vi "Client Input Test.vi"() -> (0 "error out":errorcluster, 2 "Pass?":bool)   [LabVIEW 2013, in "OPC UA Client Tests.lvlib"]
doc: "Test input override for OPC UA Client module."
uses:
  OPC UA Client Tests.lvlib
  <vilib>/NI/Tag Bus Module Framework/channel/channel classification.ctl
  module/execution/OPC UA Client runtime.lvclass
  module/execution/OPC UA Client runtime.lvclass/OPC UA Client runtime.ctl
  <vilib>/NI/Tag Bus Module Framework/channel/TBM channel.lvclass
panel:
  out "Individual Results":bool[](array[boolean])
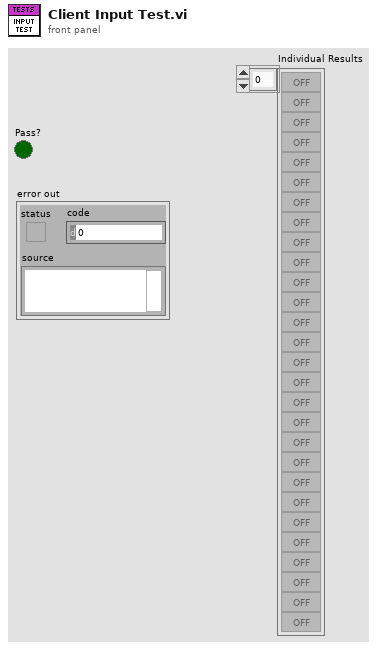
[diagram p1: front panel]
types:
  T1 = typedef "TBM channel.lvclass/channel classification.ctl" = enum16{"input data", "output data", "processing parameter", "processing result"}
  T2 = typedef "TBM channel.lvclass/data tables.ctl" = cluster{"input data":T3, "processing parameter":T3, "processing result":T3, "output data":T3}
  T3 = typedef "tag bus.lvlib/dictionary table pair.ctl" = cluster{"data dictionary":refnum<class "data dictionary.lvclass">, "data table":T4}
  T4 = typedef "tag bus.lvlib/data table.lvlib/data table.ctl" = cluster{"Double":dbl[], "Single":sgl[], "I64":i64[], "I32":i32[], "I16":i16[], "I8":i8[], "U64":u64[], "U32":u32[], "U16":u16[], "U8":u8[], "Boolean":bool[], "String":string[], "Array of Double":cluster{"DBL Array":dbl[]}[], "Array of Single":cluster{"SGL Array":sgl[]}[], "Array of I64":cluster{"I64 Array":i64[]}[], "Array of I32":cluster{"I32 Array":i32[]}[], "Array of I16":cluster{"I16 Array":i16[]}[], "Array of I8":cluster{"I8 Array":i8[]}[], "Array of U64":cluster{"U64 Array":u64[]}[], "Array of U32":cluster{"U32 Array":u32[]}[], "Array of U16":cluster{"U16 Array":u16[]}[], "Array of U8":cluster{"U8 Array":u8[]}[], "Array of Boolean":cluster{"Boolean Array":bool[]}[], "Array of String":cluster{"String Array":string[]}[]}
  T5 = typedef "OPC UA Client configuration.lvclass/Line.ctl" = cluster{"channel":refnum<class "TBM channel.lvclass">, "Node Path":string, "OPC UA Data Type":T6}
  T6 = typedef "OPC UA Client configuration.lvclass/OPC UA Data Type.ctl" = u16
  T7 = cluster{"Node Path":string, "Flattened Data":string}[]
  T8 = typedef "tag bus.lvlib/tag descriptor.lvclass/Data Type.ctl" = enum16{"Double", "Single", "I64", "I32", "I16", "I8", "U64", "U32", "U16", "U8", "Boolean", "String", "Array of Double", "Array of Single", "Array of I64", "Array of I32", "Array of I16", "Array of I8", "Array of U64", "Array of U32", "Array of U16", "Array of U8", "Array of Boolean", "Array of String"}
  T9 = cluster{"DCAF Data Type":T8, "Index":i32, "Node Path":string, "OPC UA Data Type":T6}[]
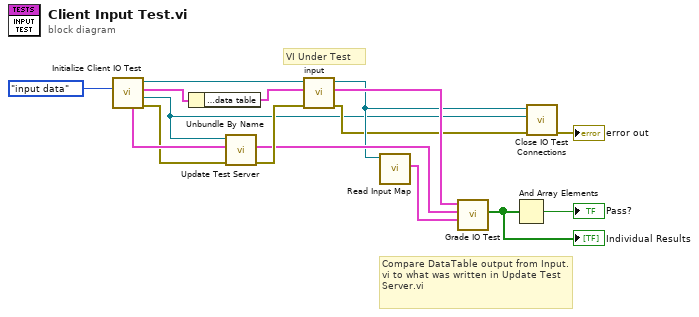
[diagram p0: block diagram]
diagram:
  # "Compare DataTable output from Input.vi to what was written in Update Test Server.vi"
  # "VI Under Test"
  n1 = call "Initialize Client IO Test.vi"("channel classification"=channel_classification."input data") -> ("error out"=w13:errorcluster, "OPC UA server refnum out"=w3:refnum<k21>, "data allocations"=w2:T2, "OPC UA runtime out"=w15:refnum<class "OPC UA Client runtime.lvclass">, "Lines"=w14:T5[])  [unwired: 6 in]
  n2 = Unbundle By Name(w2) -> ("input data.data table"=w1:T4)
  n3 = call "Update Test Server.vi"("error in (no error)"=w13, "Lines"=w14, "OPC UA server refnum in"=w3) -> ("error out"=w12:errorcluster, "Server Data"=w11:T7)  [unwired: 7 in]
  n4 = call-dynamic "input.vi"("error in"=w12, "data table in"=w1, "OPC UA runtime in"=w15) -> ("error out"=w5:errorcluster, "data table out"=w10:T4, "OPC UA runtime out"=w9:refnum<class "OPC UA Client runtime.lvclass">)  [unwired: 6 in]
  n5 = call "Read Input Map.vi"("OPC UA Client runtime in"=w9) -> ("Input Map"=w8:T9)  [unwired: 9 in, 1 out]
  n6 = call "Grade IO Test.vi"("Data Map"=w8, "Server Data"=w11, "data table in"=w10) -> ("Pass?"=w7:bool[])  [unwired: 7 in]
  "Individual Results" <- w7
  n7 = And Array Elements(Boolean array=w7) -> (logical AND=→"Pass?":bool)
  n8 = call "Close IO Test Connections.vi"("error in"=w5, "OPC UA server refnum"=w3, "OPC UA runtime in"=w9) -> ("error out"=→"error out":errorcluster)  [unwired: 8 in]
